vi "제목없음 4.vi"   [LabVIEW 2015]
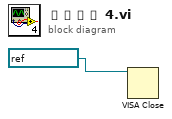
[diagram p0: block diagram]
diagram:
  n1 = VISA Close(VISA resource name=refnum<visa-resource-name> "COM10" ("Port-set 1")) -> ()  [unwired: 1 in, 1 out]
